vi "create nufern logistics xmit string.vi"(8 "error in (no error)":errorcluster, 10 "Logistics Operation":T1 {"Current RS-485 \nAddress" format="0x%02x"; "Desired RS-485 \nAddress" format="0x%02x"; "Logistics" format="0x%x" items=["Set RS-485 Address"=65, "Get RS-485 Address"=66]}, 11 "PAPA Address":i8=10 format="0x%02x") -> (0 "error out":errorcluster, 1 "String out":string, 2 "CRC Out":i32, 3 "String Out to nufern":string)   [LabVIEW 2016]
uses:
  Logistics Control 2.ctl
  2 digit hex indicator.ctl
panel:
  out "Logistics Decimal":u16
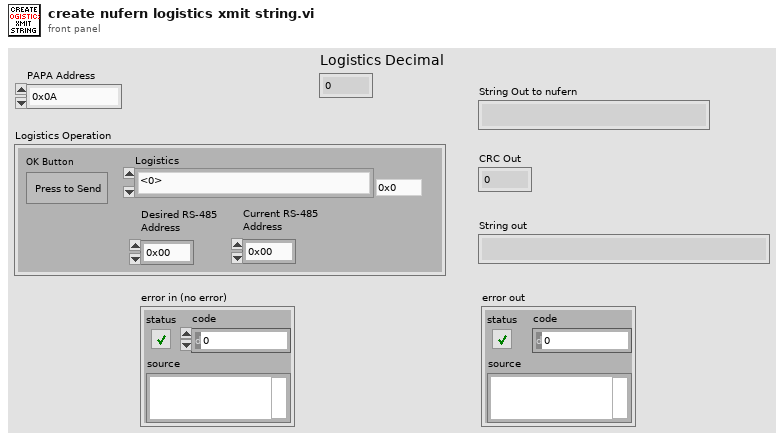
[diagram p1: front panel]
types:
  T1 = typedef "Logistics Control 2.ctl" = cluster{"Logistics":u16, "OK Button":bool, "Desired RS-485 \nAddress ":T2, "Current RS-485 \nAddress ":T2}
  T2 = typedef "2 digit hex indicator.ctl" = i32
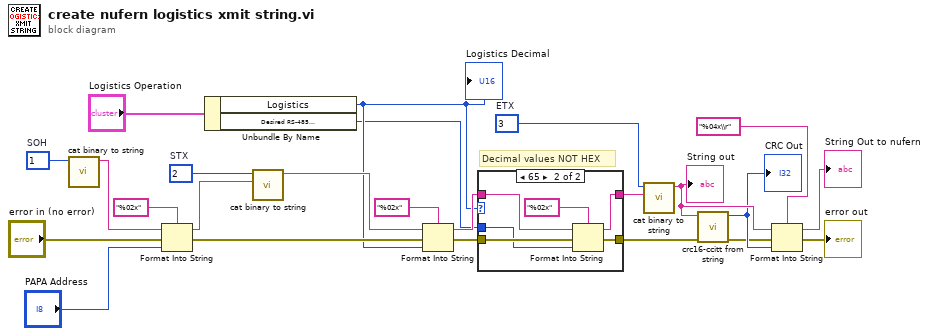
[diagram p0: block diagram]
diagram:
  w13 = 3  # ETX
  w19 = 2  # STX
  w21 = 1  # SOH
  # "Decimal values NOT HEX"
  n1 = call "cat binary to string.vi"("ETX"=w21) -> ("String out"=w22:string)  [unwired: 10 in]
  n2 = Format Into String(format string="%02x", initial string=w22, error in="error in (no error)", "PAPA Address") -> (resulting string=w18:string, error out=w16:errorcluster)
  n3 = Unbundle By Name("Logistics Operation") -> ("Logistics"=w5:u16, "Desired RS-485 \nAddress"=w1:T2)
  "Logistics Decimal" <- w5
  n4 = call "cat binary to string.vi"("String in"=w18, "ETX"=w19) -> ("String out"=w20:string)  [unwired: 9 in]
  n5 = Format Into String(format string="%02x", initial string=w20, error in=w16, w5) -> (resulting string=w6:string, error out=w3:errorcluster)
  n6 = case shown="65" w5 {
    tunnel: w6 -> [w26 w32]
    tunnel: [w26 w28] -> w4
    tunnel: w3 -> [w25 w30]
    tunnel: [w25 w29] -> w2
    tunnel: w1 -> [_ w27]
    frame 0, 66, Default {
    }
    frame 65 {
      n7 = Format Into String(format string="%02x", initial string=w32, error in=w30, w27) -> (resulting string=w28:string, error out=w29:errorcluster)
    }
  }
  n8 = call "cat binary to string.vi"("String in"=w4, "ETX"=w13) -> ("String out"=w24:string)  [unwired: 9 in]
  "String out" <- w24
  n9 = call "crc16-ccitt from string.vi"("error in (no error)"=w2, "String"=w24) -> ("error out"=w14:errorcluster, "CRC Out"=w15:i32)  [unwired: 8 in]
  "CRC Out" <- w15
  n10 = Format Into String(format string="%04x\\r", initial string=w24, error in=w14, w15) -> (resulting string=→"String Out to nufern":string, error out=→"error out":errorcluster)
